vi "CheckDuplicateData.vi"(8 "error in (no error)":errorcluster, 10 "ToCheck in":refnum<data-value>, 11 "SudukuState in":refnum<class "SudokuState.lvclass">) -> (0 "error out":errorcluster, 1 "IsDuplicate":bool, 2 "ToCheck out":refnum<data-value>, 3 "SudukuState out":refnum<class "SudokuState.lvclass">)   [LabVIEW 2013, in "SudokuState.lvclass"]
uses:
  SudokuState.lvclass
  LLNode/LLNode.lvclass
  SudokuState.lvclass/SudokuState.ctl
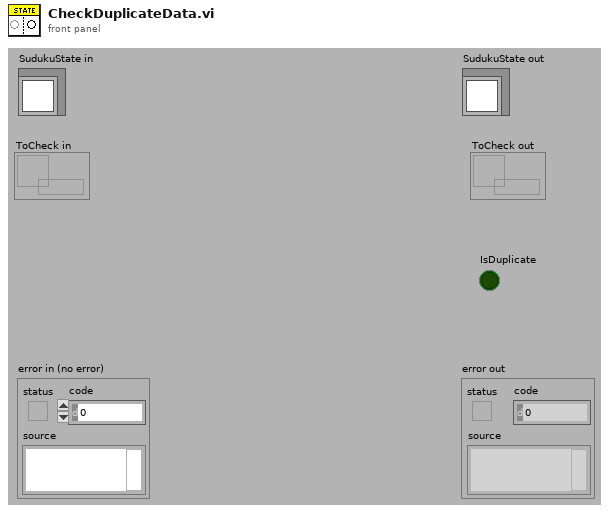
[diagram p1: front panel]
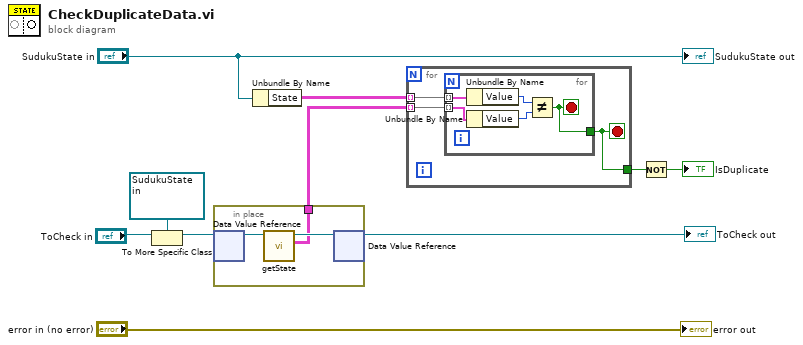
[diagram p0: block diagram]
diagram:
  n1 = To More Specific Class(target class=refnum<data-value> refnum ("data value reference"), reference="ToCheck in") -> (specific class reference=w8:refnum<data-value>)  [unwired: 1 in, 1 out]
  n2 = in-place {
    in-place-border: [w11] -> w5
    n3 = in-place-dvr #1(w8) -> (w13:refnum<class "SudokuState.lvclass">)  [unwired: 1 out]
    n4 = call "getState.vi"("SudukuState in"=w13) -> ("State"=w11:cluster{"Value":i32, "Options":i32[]}[][], "SudukuState out"=w12:refnum<class "SudokuState.lvclass">)  [unwired: 8 in, 1 out]
    n5 = in-place-dvr #1(w12) -> (→"ToCheck out":refnum<data-value>)  [unwired: 1 out]
  }
  n6 = Unbundle By Name("SudukuState in") -> ("State"=w6:cluster{"Value":i32, "Options":i32[]}[][])
  n7 = for {
    tunnel: w6 -> [w16] mode=indexing
    tunnel: w5 -> [w15] mode=indexing
    tunnel: [w14] -> w2
    stop <- w14 stop-if-true
    n8 = for {
      tunnel: w16 -> [w21] mode=indexing
      tunnel: w15 -> [w20] mode=indexing
      tunnel: [w17] -> w14
      stop <- w17 stop-if-true
      n9 = Unbundle By Name(w21) -> ("Value"=w19:i32)
      n10 = Unbundle By Name(w20) -> ("Value"=w18:i32)
      n11 = Not Equal?(x=w19, y=w18) -> (x != y?=w17:bool)
    }
  }
  n12 = Not(x=w2) -> (.not. x?=→"IsDuplicate":bool)
  "error out" <- "error in (no error)"
  "SudukuState out" <- "SudukuState in"
